vi "Add Items by Text ImageIndex Array and SubItems to ListView.vi"(7 "SubItems":string[][](array[string]), 8 "error in (no error)":errorcluster caption="错误输入（无错误）", 9 "ImageIndex":i32[](array[numeric]), 10 "Text":string[](array[string]), 11 "ListViewClass 输入":refnum<class "ListViewClass.lvclass"> caption="DNL_LabVIEW Object in") -> (0 "error out":errorcluster caption="错误输出", 3 "ListViewClass 输出":refnum<class "ListViewClass.lvclass"> caption="DNL_LabVIEW Object out")   [LabVIEW 2012, in "ListViewClass.lvclass"]
uses:
  ListViewClass.lvclass
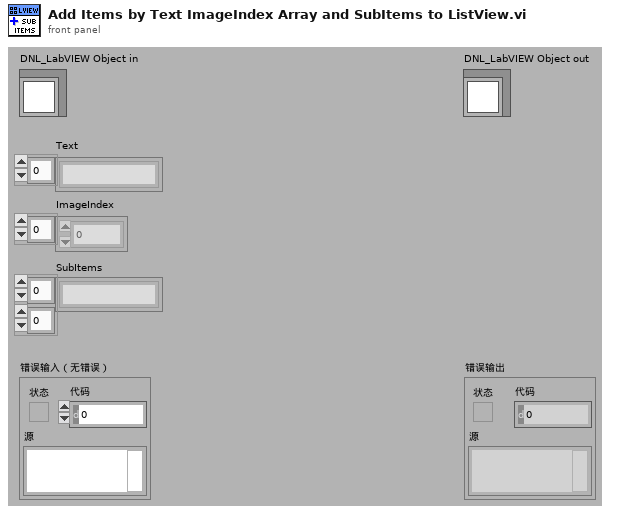
[diagram p1: front panel]
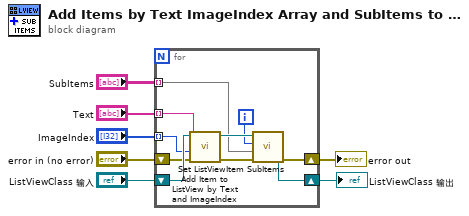
[diagram p0: block diagram]
diagram:
  n1 = for {
    shift-right: [w10] -> w2
    shift-left: "ListViewClass 输入" -> [w17]
    tunnel: "Text" -> [w16] mode=indexing
    tunnel: "ImageIndex" -> [w15] mode=indexing
    tunnel: "SubItems" -> [w11] mode=indexing
    shift-right: [w8] -> w1
    shift-left: "error in (no error)" -> [w9]
    i -> [w12]
    n2 = call "Add Item to ListView by Text and ImageIndex.vi"("error in (no error)"=w9, "imageIndex"=w15, "text"=w16, "ListViewClass 输入"=w17) -> ("error out"=w13:errorcluster, "ListViewClass 输出"=w14:refnum<class "ListViewClass.lvclass">)  [unwired: 6 in]
    n3 = call "Set ListViewItem SubItems.vi"("error in (no error)"=w13, "SubItems"=w11, "index"=w12, "ListViewClass 输入"=w14) -> ("error out"=w8:errorcluster, "ListViewClass 输出"=w10:refnum<class "ListViewClass.lvclass">)  [unwired: 6 in]
  }
  "error out" <- w1
  "ListViewClass 输出" <- w2
